vi "Multiple Image Stitching LV 86.vi"() -> ()   [LabVIEW 2017]
uses:
  <vilib>/vision/NI_Vision_Development_Module.lvlib
panel:
  out "Image 4":T1(plugin-control)
  out "Image 3":T1(plugin-control)
  out "Stiched Image":T1(plugin-control)
  out "Image 2":T1(plugin-control)
  out "Image 1":T1(plugin-control)
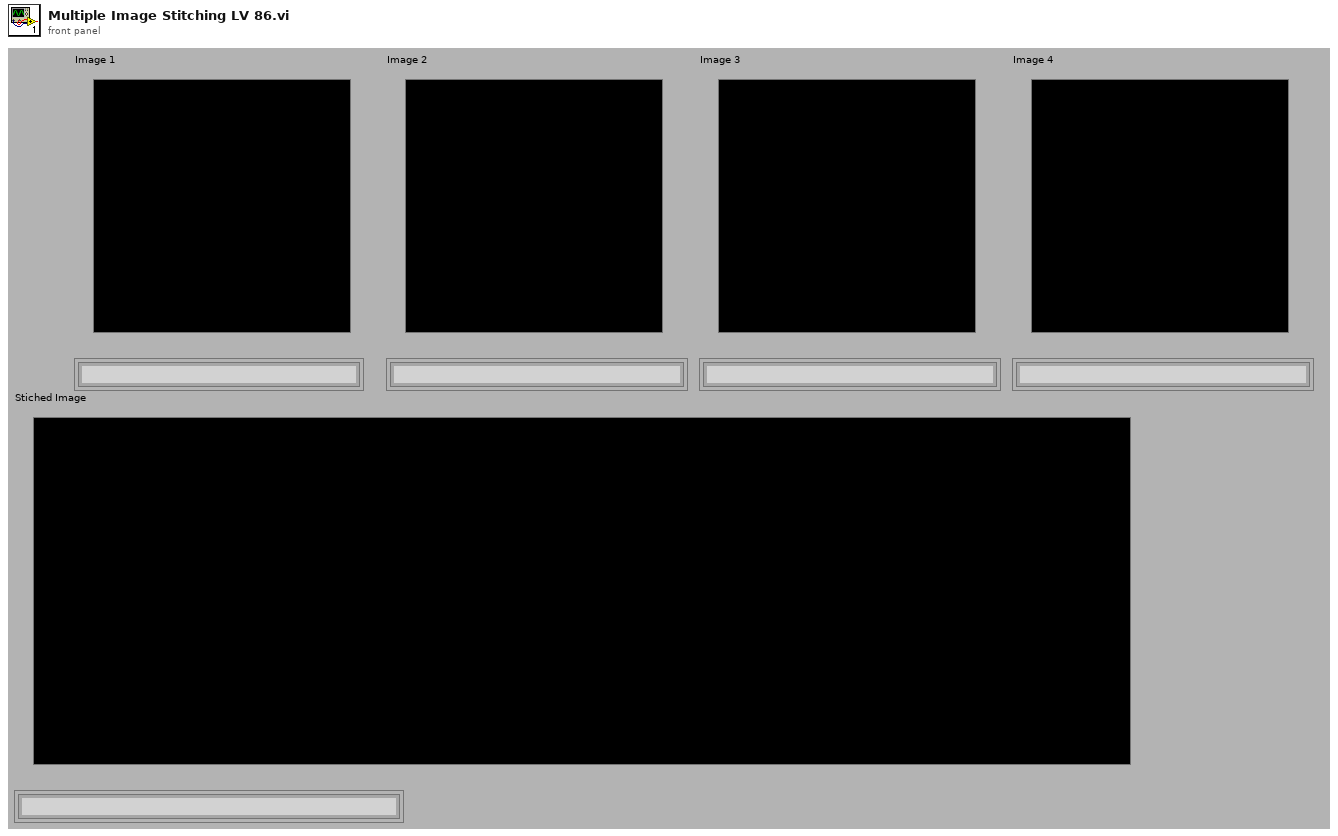
[diagram p1: front panel]
types:
  T1 = typedef "IMAQ Image.ctl" = refnum<image>
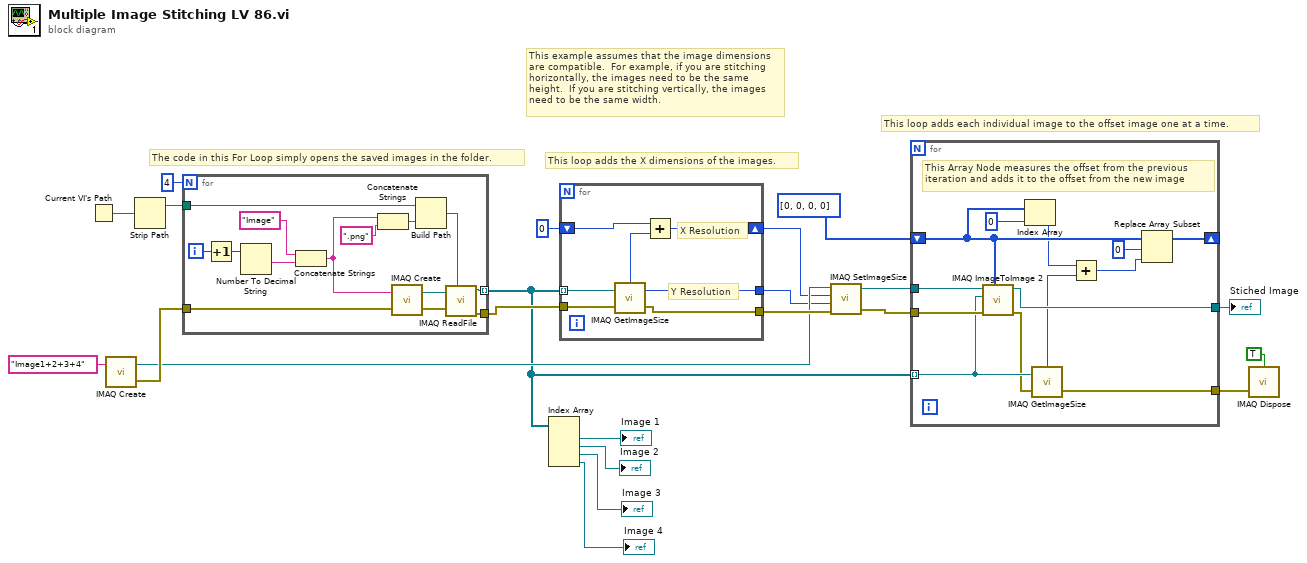
[diagram p0: block diagram]
diagram:
  # "This loop adds each individual image to the offset image one at a time."
  # "This loop adds the X dimensions of the images."
  # "This example assumes that the image dimensions\nare compatible.  For example, if you are stitching\nhorizontally, the images need to be the same\nheight.  If you are stitching vertically, the images\nneed to be the same width."
  # "The code in this For Loop simply opens the saved images in the folder."
  n1 = Current VI's Path() -> (path=w21:path)
  n2 = call "IMAQ Create"("Image Name"="Image1+2+3+4") -> ("New Image"=w14:T1, "error out"=w19:errorcluster)  [unwired: 3 in, 1 out]
  n3 = Strip Path(path=w21) -> (stripped path=w20:path)  [unwired: 1 out]
  n4 = for {
    N: 4 -> [_]
    tunnel: w20 -> [w34]
    tunnel: [w28] -> w7 mode=indexing
    tunnel: [w27] -> w16
    tunnel: w19 -> [w26]
    i -> [w33]
    n5 = Increment(x=w33) -> (x+1=w32:i32)
    n6 = Number To Decimal String(number=w32) -> (decimal integer string=w36:string)  [unwired: 1 out]
    n7 = Concatenate Strings("Image", w36) -> (w23:string)
    n8 = Concatenate Strings(w23, ".png") -> (w25:string)
    n9 = call "IMAQ Create"("Image Name"=w23, "error in (no error)"=w26) -> ("New Image"=w30:T1, "error out"=w31:errorcluster)  [unwired: 2 in, 1 out]
    n10 = Build Path(base path=w34, name or relative path=w25) -> (appended path=w29:path)
    n11 = call "IMAQ ReadFile"("File Path"=w29, "error in (no error)"=w31, "Image"=w30) -> ("error out"=w27:errorcluster, "Image Out"=w28:T1)  [unwired: 2 in, 5 out]
  }
  n12 = Index Array(array=w7) -> (element #1=→"Image 1":T1, element #2=→"Image 2":T1, element #3=→"Image 3":T1, element #4=→"Image 4":T1)  [unwired: 4 in]
  n13 = for {
    tunnel: w7 -> [w43] mode=indexing
    shift-right: [w41] -> w13
    shift-left: 0 ("Y Resolution") -> [w42]
    tunnel: w16 -> [w40]
    tunnel: [w39] -> w12
    tunnel: [w38] -> w15
    # "Y Resolution"
    # "X Resolution"
    n14 = call "IMAQ GetImageSize"("Image"=w43, "error in (no error)"=w40) -> ("Y Resolution"=w39:i32, "X Resolution"=w37:i32, "error out"=w38:errorcluster)  [unwired: 2 out]
    n15 = Add(x=w42, y=w37) -> (x+y=w41:i32)
  }
  n16 = call "IMAQ SetImageSize"("error in (no error)"=w15, "Y Resolution"=w12, "X Resolution"=w13, "Image"=w14) -> ("error out"=w10:errorcluster, "Image Out"=w11:T1)  [unwired: 1 out]
  n17 = for {
    tunnel: w7 -> [w53] mode=indexing
    tunnel: w11 -> [w54]
    tunnel: w10 -> [w56]
    tunnel: [w55] -> w8
    shift-right: [w52] -> _
    shift-left: i32[] [0, 0, 0, 0] -> [w47]
    tunnel: [w50] -> w4
    # "This Array Node measures the offset from the previous\niteration and adds it to the offset from the new image"
    n18 = call "IMAQ ImageToImage 2"("Offset Left/Top"=w47, "error in (no error)"=w56, "Image Src (Small)"=w53, "Image Src (Large)"=w54) -> ("error out"=w51:errorcluster, "Image Dst Out"=w55:T1)  [unwired: 2 in, 4 out]
    n19 = Index Array(array=w47, index=0) -> (element=w46:i32)
    n20 = call "IMAQ GetImageSize"("Image"=w53, "error in (no error)"=w51) -> ("X Resolution"=w45:i32, "error out"=w50:errorcluster)  [unwired: 3 out]
    n21 = Add(x=w46, y=w45) -> (x+y=w44:i32)
    n22 = Replace Array Subset(array=w47, new element=w44, index=0) -> (w52:i32[])
  }
  "Stiched Image" <- w8
  n23 = call "IMAQ Dispose"("All Images? (No)"=TRUE, "error in (no error)"=w4) -> ()  [unwired: 1 in, 4 out]
